vi "Severity - name round trip.vi"(8 "error in (no error)":errorcluster) -> (0 "error out":errorcluster)   [LabVIEW 2026, in "Tests.lvlib"]
doc: "Unit test (Caraya). Verifies the Severity name mapping round-trips and that an unknown name faults: enum-to-name for FATAL/INFO/ALL, name-to-enum for FATAL/TRACE/OFF including the OFF and ALL sentinels, and SeverityFromString returning an error on an unrecognized name (SRS-LMBR-048, R5). Pure, no fixtures."
uses:
  Tests.lvlib
  src/TypeDefs/Severity.ctl
  <vilib>/addons/_JKI Toolkits/Caraya/classes/Assert/Assert Equal Value_Variant.vi
  <vilib>/addons/_JKI Toolkits/Caraya/classes/Assert/Assert Error.vi
  <vilib>/addons/_JKI Toolkits/Caraya/classes/Test/Test.lvclass
  src/Lumberjack.lvlib
  <vilib>/addons/_JKI Toolkits/Caraya/classes/Assert/Assert.lvclass
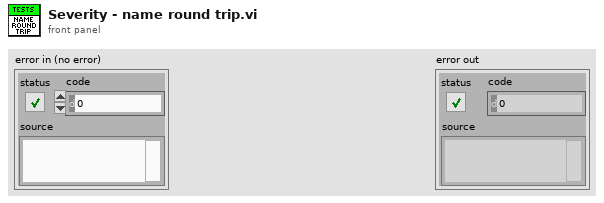
[diagram p1: front panel]
types:
  T1 = typedef "Lumberjack.lvlib/Severity.ctl" = enum16{"OFF", "FATAL", "ERROR", "WARN", "INFO", "DEBUG", "TRACE", "ALL"}
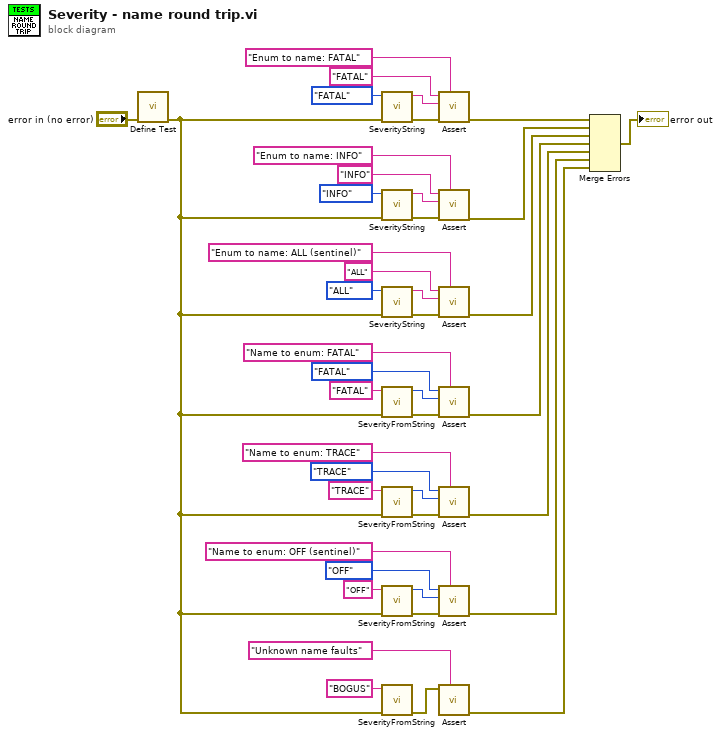
[diagram p0: block diagram]
diagram:
  n1 = call <vilib>:"Define Test.vi"("error in (no error)"="error in (no error)") -> ("error out"=w5:errorcluster)  [unwired: 9 in, 1 out]
  n2 = call "SeverityString.vi"("error in (no error)"=w5, "Severity"=Severity."FATAL") -> ("error out"=w42:errorcluster, "SeverityString"=w41:string)  [unwired: 8 in]
  n3 = call "SeverityString.vi"("error in (no error)"=w5, "Severity"=Severity."INFO") -> ("error out"=w37:errorcluster, "SeverityString"=w36:string)  [unwired: 8 in]
  n4 = call "SeverityString.vi"("error in (no error)"=w5, "Severity"=Severity."ALL") -> ("error out"=w29:errorcluster, "SeverityString"=w28:string)  [unwired: 8 in]
  n5 = call "SeverityFromString.vi"("error in (no error)"=w5, "SeverityString"="FATAL") -> ("error out"=w23:errorcluster, "Severity"=w19:T1)  [unwired: 8 in]
  n6 = call "SeverityFromString.vi"("error in (no error)"=w5, "SeverityString"="TRACE") -> ("error out"=w18:errorcluster, "Severity"=w14:T1)  [unwired: 8 in]
  n7 = call "SeverityFromString.vi"("error in (no error)"=w5, "SeverityString"="OFF") -> ("error out"=w13:errorcluster, "Severity"=w9:T1)  [unwired: 8 in]
  n8 = call "SeverityFromString.vi"("error in (no error)"=w5, "SeverityString"="BOGUS") -> ("error out"=w6:errorcluster)  [unwired: 8 in, 1 out]
  n9 = call-poly <vilib>:"Assert.vi"("Label"="Enum to name: FATAL", "error in (no error)"=w42, "Actual"=w41, "Expected"="FATAL") -> ("error out"=w32:errorcluster)  [unwired: 6 in, 1 out]
  n10 = call-poly <vilib>:"Assert.vi"("Label"="Enum to name: INFO", "error in (no error)"=w37, "Actual"=w36, "Expected"="INFO") -> ("error out"=w30:errorcluster)  [unwired: 6 in, 1 out]
  n11 = call-poly <vilib>:"Assert.vi"("Label"="Enum to name: ALL (sentinel)", "error in (no error)"=w29, "Actual"=w28, "Expected"="ALL") -> ("error out"=w24:errorcluster)  [unwired: 6 in, 1 out]
  n12 = call-poly <vilib>:"Assert.vi"("Label"="Name to enum: FATAL", "error in (no error)"=w23, "Actual"=w19, "Expected"=Severity."FATAL" ("Severity")) -> ("error out"=w4:errorcluster)  [unwired: 6 in, 1 out]
  n13 = call-poly <vilib>:"Assert.vi"("Label"="Name to enum: TRACE", "error in (no error)"=w18, "Actual"=w14, "Expected"=Severity."TRACE" ("Severity")) -> ("error out"=w3:errorcluster)  [unwired: 6 in, 1 out]
  n14 = call-poly <vilib>:"Assert.vi"("Label"="Name to enum: OFF (sentinel)", "error in (no error)"=w13, "Actual"=w9, "Expected"=Severity."OFF" ("Severity")) -> ("error out"=w2:errorcluster)  [unwired: 6 in, 1 out]
  n15 = call-poly <vilib>:"Assert.vi"("Label"="Unknown name faults", "Error?"=w6) -> ("error out"=w1:errorcluster)  [unwired: 8 in, 1 out]
  n16 = Merge Errors(w32, w30, w24, w4, w3, w2, w1) -> (→"error out":errorcluster)
